vi "Teleop.vi"(10 "Match Info":T1={"Autonomous Elapsed Seconds"=0.0, "TeleOp Elapsed Seconds"=0.0, "Disabled Elapsed Seconds"=0.0, "Visited Autonomous"=FALSE, "Visited TeleOp"=FALSE, "Visited Disabled"=FALSE, "Autonomous Settings"={"Autonomous Style"=enum."Independent", "VI Refnum"=refnum}}, 11 "Call Context":T2) -> ()   [LabVIEW 2017]
doc: "This VI is called for each enabled TeleOp packet received from the DS. It is typically used to read from joysticks and other inputs and update I/O or setpoints for timed control loops. It should complete and return within 20 milliseconds or risk missing DS packets."
uses:
  <vilib>/Rock Robotics/WPI/DriverStation/WPI_DriverStationDerivedRobotMode.ctl
  <vilib>/Rock Robotics/WPI/DriverStation/WPI_DriverStationMatch Info.ctl
  Framework/Robot Global Data.vi
panel:
  out "Hardware Fault":bool
  out "Temperature Fault":bool
  out "Battery Voltage Fault":bool
  out "Current Faults":bool[](array[boolean])
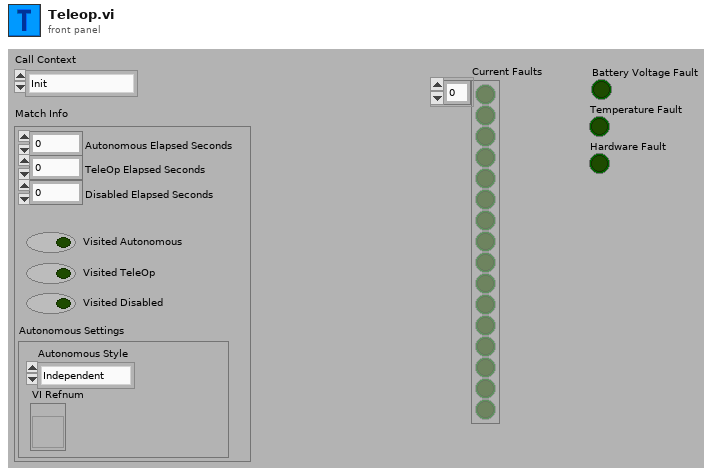
[diagram p1: front panel]
types:
  T1 = typedef "WPI_DriverStationMatch Info.ctl" = cluster{"Autonomous Elapsed Seconds":dbl, "TeleOp Elapsed Seconds":dbl, "Disabled Elapsed Seconds":dbl, "Visited Autonomous":bool, "Visited TeleOp":bool, "Visited Disabled":bool, "Autonomous Settings":cluster{"Autonomous Style":enum16{"Iterative", "Independent"}, "VI Refnum":refnum<vi>}}
  T2 = typedef "WPI_DriverStationDerivedRobotMode.ctl" = enum16{"Init", "Execute", "Stop"}
  T3 = enum16{"Normal", "Square", "Square with Rate", "Square Root", "Linear", "Exponential"}
  T4 = enum16{"Linear", "Square  Root", "Square", "n^x"}
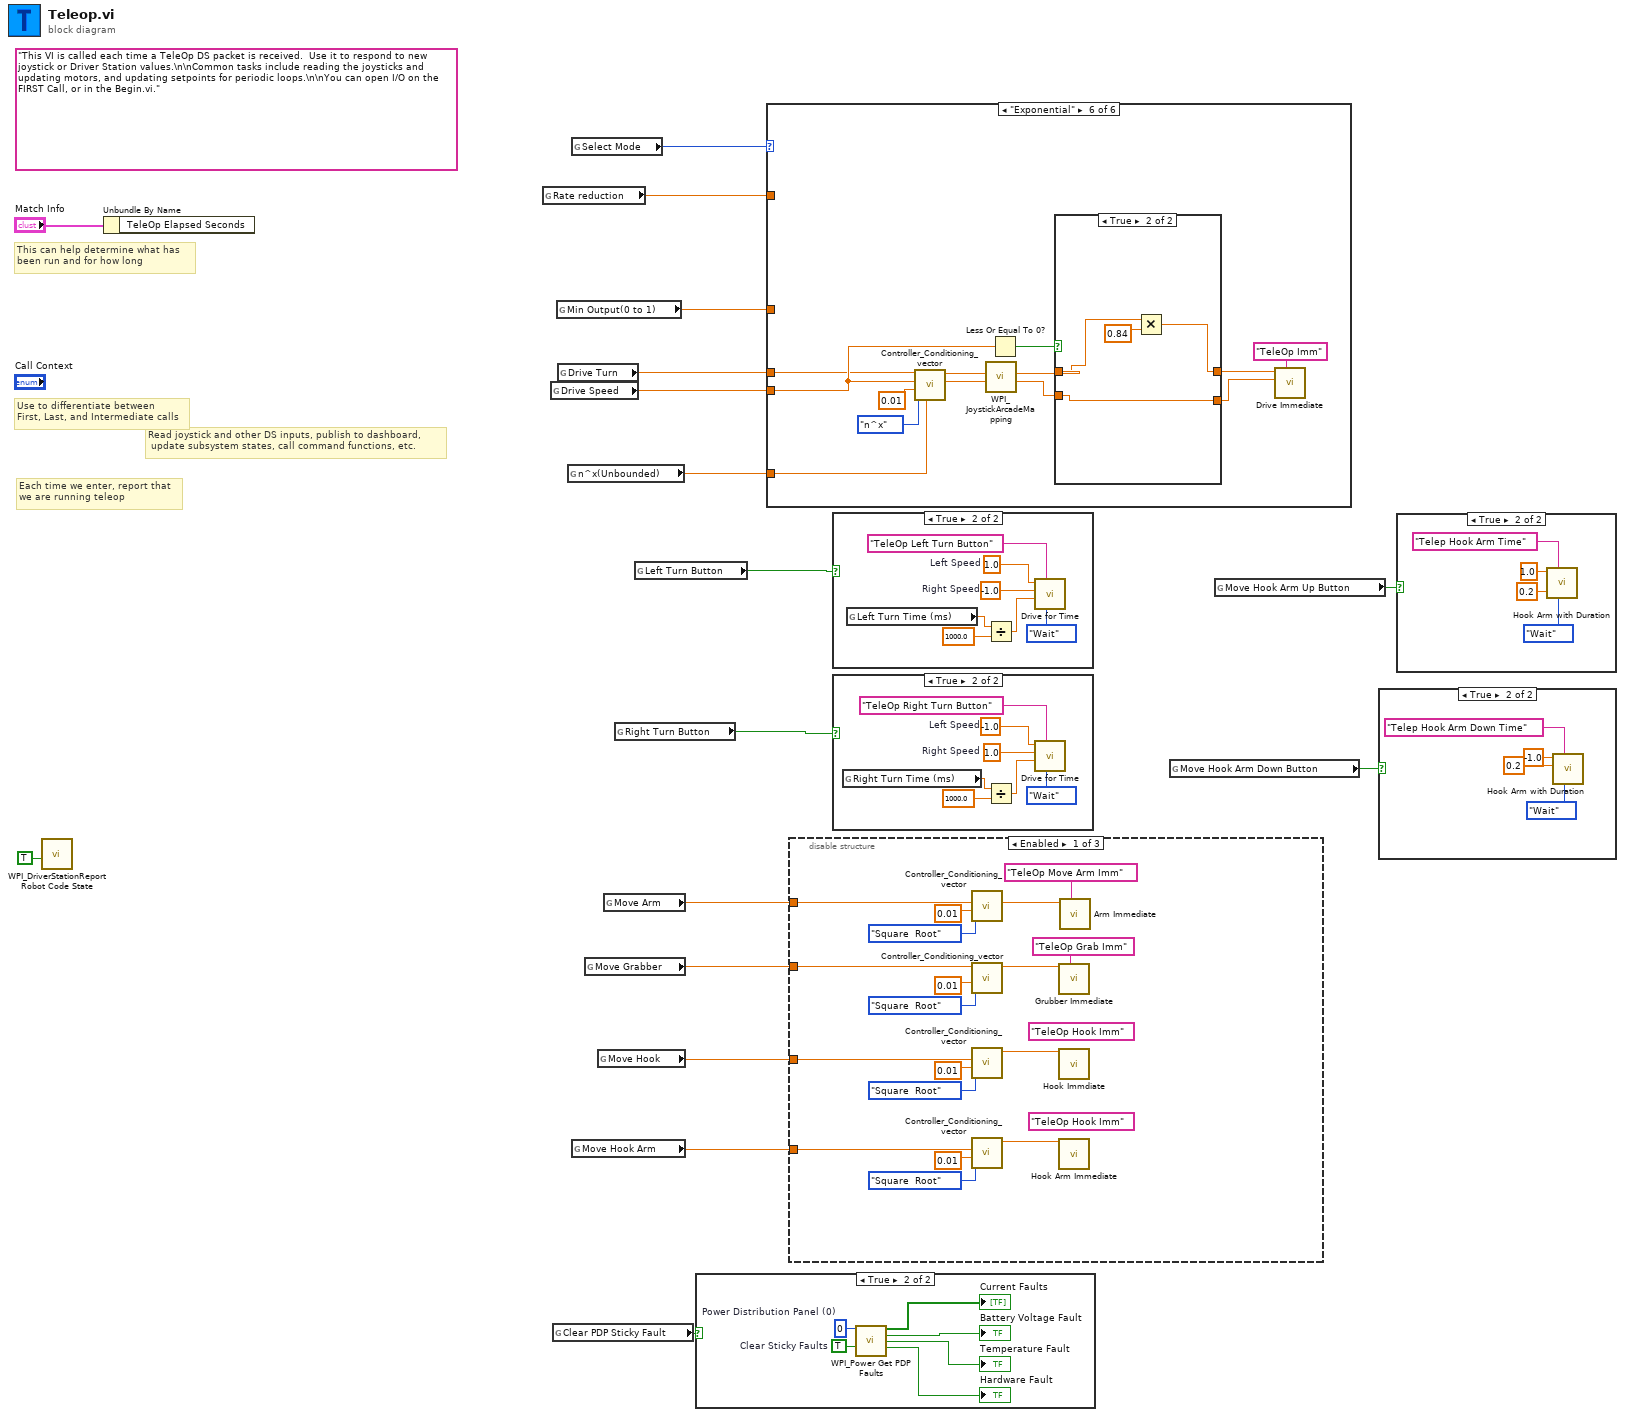
[diagram p0: block diagram]
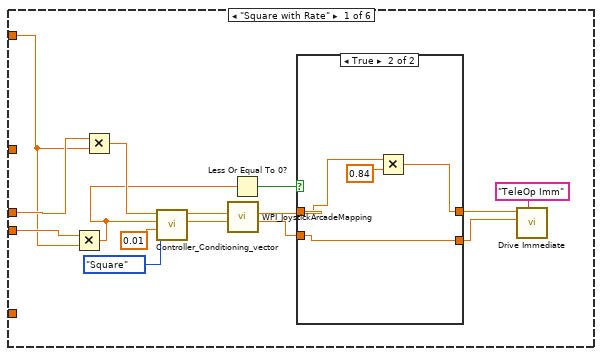
[diagram p7: hidden frame]
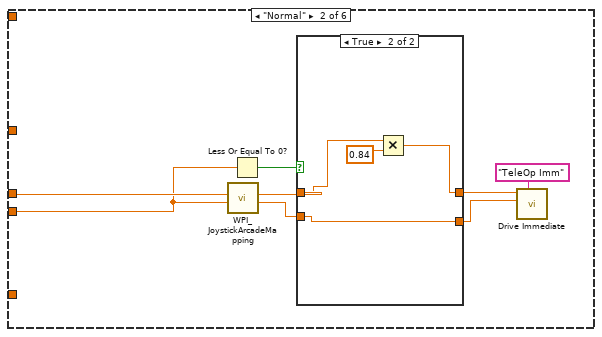
[diagram p9: hidden frame]
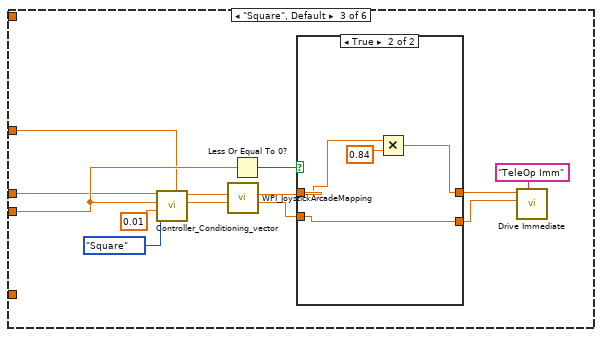
[diagram p11: hidden frame]
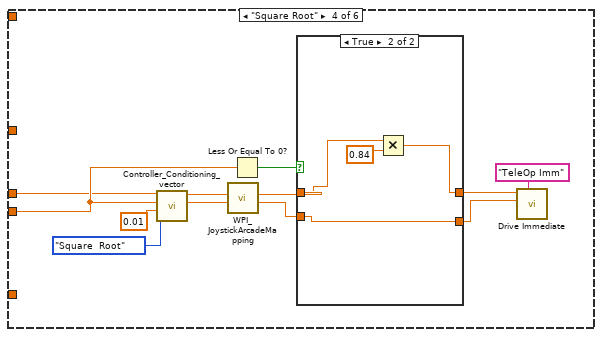
[diagram p13: hidden frame]
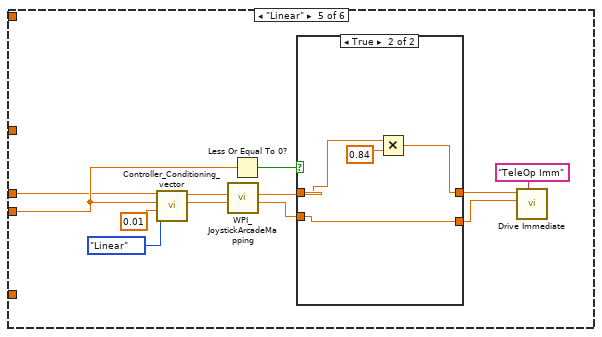
[diagram p15: hidden frame]
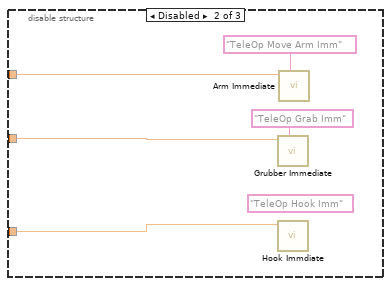
[diagram p18: hidden frame]
diagram:
  (unwired) "This VI is called each time a TeleOp DS packet is received.  Use it to respond to new joystick or Driver Station values.\n\nCommon tasks include reading the joysticks and updating motors, and updating setpoints for periodic loops.\n\nYou can open I/O on the FIRST Call, or in the Begin.vi."
  # "Read joystick and other DS inputs, publish to dashboard,\n update subsystem states, call command functions, etc."
  # "Each time we enter, report that\nwe are running teleop"
  # "Use to differentiate between\nFirst, Last, and Intermediate calls"
  # "This can help determine what has\nbeen run and for how long"
  n1 = call <vilib>:"WPI_DriverStationReport Robot Code State.vi"("TeleOp"=TRUE ("Autonomous")) -> ()  [unwired: 10 in, 1 out]
  n2 = Unbundle By Name("Match Info") -> ()  [unwired: 1 out]
  n3 = global read "Robot Global Data.vi" "Rate reduction"() -> (w12:dbl)
  n4 = global read "Robot Global Data.vi" "Drive Speed"() -> (w10:dbl)
  n5 = global read "Robot Global Data.vi" "Clear PDP Sticky Fault"() -> (w3:bool)
  n6 = global read "Robot Global Data.vi" "Min Output(0 to 1)"() -> (w14:dbl)
  n7 = global read "Robot Global Data.vi" "Drive Turn"() -> (w11:dbl)
  n8 = global read "Robot Global Data.vi" "n^x(Unbounded)"() -> (w13:dbl)
  n9 = global read "Robot Global Data.vi" "Select Mode"() -> (w15:T3)
  n10 = global read "Robot Global Data.vi" "Move Hook Arm"() -> (w4:dbl)
  n11 = global read "Robot Global Data.vi" "Move Grabber"() -> (w6:dbl)
  n12 = global read "Robot Global Data.vi" "Move Hook"() -> (w5:dbl)
  n13 = global read "Robot Global Data.vi" "Move Arm"() -> (w7:dbl)
  n14 = global read "Robot Global Data.vi" "Right Turn Button"() -> (w8:bool)
  n15 = global read "Robot Global Data.vi" "Left Turn Button"() -> (w9:bool)
  n16 = case shown="True" w3 {
    frame False {
    }
    frame True {
      w22 = TRUE  # Clear Sticky Faults
      w23 = u8 0  # Power Distribution Panel (0)
      n17 = call <vilib>:"WPI_Power Get PDP Faults.vi"("Power Distribution Panel (0)"=w23, "Clear Sticky Faults"=w22) -> ("Current Faults"=→"Current Faults":bool[], "Battery Voltage Fault"=→"Battery Voltage Fault":bool, "Temperature Fault"=→"Temperature Fault":bool, "Hardware Fault"=→"Hardware Fault":bool)  [unwired: 9 in, 1 out]
    }
  }
  n18 = case shown="\"Exponential\"" w15 {
    tunnel: w11 -> [w38 w46 w60 w78 w96 w115]
    tunnel: w10 -> [w37 w45 w61 w79 w97 w116]
    tunnel: w14 -> [_ _ w59 _ _ _]
    tunnel: w13 -> [_ _ _ _ _ w114]
    tunnel: w12 -> [w24 _ _ _ _ _]
    frame "Square with Rate" {
      n19 = Multiply(x=w37, y=w24) -> (x*y=w25:dbl)
      n20 = Multiply(x=w38, y=w24) -> (x*y=w26:dbl)
      n21 = call "Controller_Conditioning_vector.vi"("Enum"=T4."Square", "Dead Zone(0 to 1)"=0.01, "Y(-1 to 1)"=w25, "X(-1 to 1)"=w26) -> ("Y"=w27:dbl, "X"=w28:dbl)  [unwired: 4 in, 2 out]
      n22 = call <vilib>:"WPI_JoystickArcadeMapping.vi"("Y axis value"=w27, "X axis value"=w28) -> ("Right Motor Value"=w33:dbl, "Left Motor Value"=w34:dbl)  [unwired: 8 in]
      n23 = Less Or Equal To 0?(x=w25) -> (x <= 0?=w35:bool)
      n24 = case shown="True" w35 {
        tunnel: w34 -> [w39 w43]
        tunnel: [w39 w42] -> w32
        tunnel: w33 -> [w40 w41]
        tunnel: [w40 w41] -> w31
        frame False {
        }
        frame True {
          n25 = Multiply(x=w43, y=0.84) -> (x*y=w42:dbl)
        }
      }
      n26 = call "Drive Immediate.vi"("Description"="TeleOp Imm", "Right Setpoint"=w31, "Left Setpoint"=w32) -> ()  [unwired: 8 in, 1 out]
    }
    frame "Normal" {
      n27 = call <vilib>:"WPI_JoystickArcadeMapping.vi"("Y axis value"=w45, "X axis value"=w46) -> ("Right Motor Value"=w49:dbl, "Left Motor Value"=w50:dbl)  [unwired: 8 in]
      n28 = Less Or Equal To 0?(x=w45) -> (x <= 0?=w51:bool)
      n29 = case shown="True" w51 {
        tunnel: w50 -> [w53 w57]
        tunnel: [w53 w56] -> w48
        tunnel: w49 -> [w54 w55]
        tunnel: [w54 w55] -> w47
        frame False {
        }
        frame True {
          n30 = Multiply(x=w57, y=0.84) -> (x*y=w56:dbl)
        }
      }
      n31 = call "Drive Immediate.vi"("Description"="TeleOp Imm", "Right Setpoint"=w47, "Left Setpoint"=w48) -> ()  [unwired: 8 in, 1 out]
    }
    frame "Square", Default {
      n32 = call "Controller_Conditioning_vector.vi"("Min Output(0 to 1)"=w59, "Enum"=T4."Square", "Dead Zone(0 to 1)"=0.01, "Y(-1 to 1)"=w61, "X(-1 to 1)"=w60) -> ("Y"=w62:dbl, "X"=w63:dbl)  [unwired: 3 in, 2 out]
      n33 = call <vilib>:"WPI_JoystickArcadeMapping.vi"("Y axis value"=w62, "X axis value"=w63) -> ("Right Motor Value"=w68:dbl, "Left Motor Value"=w69:dbl)  [unwired: 8 in]
      n34 = Less Or Equal To 0?(x=w61) -> (x <= 0?=w70:bool)
      n35 = case shown="True" w70 {
        tunnel: w69 -> [w72 w76]
        tunnel: [w72 w75] -> w67
        tunnel: w68 -> [w73 w74]
        tunnel: [w73 w74] -> w66
        frame False {
        }
        frame True {
          n36 = Multiply(x=w76, y=0.84) -> (x*y=w75:dbl)
        }
      }
      n37 = call "Drive Immediate.vi"("Description"="TeleOp Imm", "Right Setpoint"=w66, "Left Setpoint"=w67) -> ()  [unwired: 8 in, 1 out]
    }
    frame "Square Root" {
      n38 = call "Controller_Conditioning_vector.vi"("Enum"=T4."Square  Root", "Dead Zone(0 to 1)"=0.01, "Y(-1 to 1)"=w79, "X(-1 to 1)"=w78) -> ("Y"=w80:dbl, "X"=w81:dbl)  [unwired: 4 in, 2 out]
      n39 = call <vilib>:"WPI_JoystickArcadeMapping.vi"("Y axis value"=w80, "X axis value"=w81) -> ("Right Motor Value"=w86:dbl, "Left Motor Value"=w87:dbl)  [unwired: 8 in]
      n40 = Less Or Equal To 0?(x=w79) -> (x <= 0?=w88:bool)
      n41 = case shown="True" w88 {
        tunnel: w87 -> [w90 w94]
        tunnel: [w90 w93] -> w85
        tunnel: w86 -> [w91 w92]
        tunnel: [w91 w92] -> w84
        frame False {
        }
        frame True {
          n42 = Multiply(x=w94, y=0.84) -> (x*y=w93:dbl)
        }
      }
      n43 = call "Drive Immediate.vi"("Description"="TeleOp Imm", "Right Setpoint"=w84, "Left Setpoint"=w85) -> ()  [unwired: 8 in, 1 out]
    }
    frame "Linear" {
      n44 = call "Controller_Conditioning_vector.vi"("Enum"=T4."Linear", "Dead Zone(0 to 1)"=0.01, "Y(-1 to 1)"=w97, "X(-1 to 1)"=w96) -> ("Y"=w98:dbl, "X"=w99:dbl)  [unwired: 4 in, 2 out]
      n45 = call <vilib>:"WPI_JoystickArcadeMapping.vi"("Y axis value"=w98, "X axis value"=w99) -> ("Right Motor Value"=w104:dbl, "Left Motor Value"=w105:dbl)  [unwired: 8 in]
      n46 = Less Or Equal To 0?(x=w97) -> (x <= 0?=w106:bool)
      n47 = case shown="True" w106 {
        tunnel: w105 -> [w108 w112]
        tunnel: [w108 w111] -> w103
        tunnel: w104 -> [w109 w110]
        tunnel: [w109 w110] -> w102
        frame False {
        }
        frame True {
          n48 = Multiply(x=w112, y=0.84) -> (x*y=w111:dbl)
        }
      }
      n49 = call "Drive Immediate.vi"("Description"="TeleOp Imm", "Right Setpoint"=w102, "Left Setpoint"=w103) -> ()  [unwired: 8 in, 1 out]
    }
    frame "Exponential" {
      n50 = call "Controller_Conditioning_vector.vi"("n^x(Unbounded)"=w114, "Enum"=T4."n^x", "Dead Zone(0 to 1)"=0.01, "Y(-1 to 1)"=w116, "X(-1 to 1)"=w115) -> ("Y"=w117:dbl, "X"=w118:dbl)  [unwired: 3 in, 2 out]
      n51 = call <vilib>:"WPI_JoystickArcadeMapping.vi"("Y axis value"=w117, "X axis value"=w118) -> ("Right Motor Value"=w123:dbl, "Left Motor Value"=w124:dbl)  [unwired: 8 in]
      n52 = Less Or Equal To 0?(x=w116) -> (x <= 0?=w125:bool)
      n53 = case shown="True" w125 {
        tunnel: w124 -> [w127 w131]
        tunnel: [w127 w130] -> w122
        tunnel: w123 -> [w128 w129]
        tunnel: [w128 w129] -> w121
        frame False {
        }
        frame True {
          n54 = Multiply(x=w131, y=0.84) -> (x*y=w130:dbl)
        }
      }
      n55 = call "Drive Immediate.vi"("Description"="TeleOp Imm", "Right Setpoint"=w121, "Left Setpoint"=w122) -> ()  [unwired: 8 in, 1 out]
    }
  }
  n56 = disable-structure shown="Enabled" {
    disable-tunnel: w7 -> [w145 w153 _]
    disable-tunnel: w6 -> [w144 w152 _]
    disable-tunnel: w5 -> [w137 w151 _]
    disable-tunnel: w4 -> [w136 _ _]
    frame Enabled {
      (unwired) "TeleOp Hook Imm" ("Description")
      (unwired) "TeleOp Hook Imm" ("Description")
      n57 = call "Controller_Conditioning_vector.vi"("Enum"=T4."Square  Root", "Dead Zone(0 to 1)"=0.01, "Y(-1 to 1)"=w145) -> ("Y"=w148:dbl)  [unwired: 5 in, 3 out]
      n58 = call "Controller_Conditioning_vector.vi"("Enum"=T4."Square  Root", "Dead Zone(0 to 1)"=0.01, "X(-1 to 1)"=w144) -> ("X"=w143:dbl)  [unwired: 5 in, 3 out]
      n59 = call "Controller_Conditioning_vector.vi"("Enum"=T4."Square  Root", "Dead Zone(0 to 1)"=0.01, "Y(-1 to 1)"=w137) -> ("X"=w140:dbl)  [unwired: 5 in, 3 out]
      n60 = call "Controller_Conditioning_vector.vi"("Enum"=T4."Square  Root", "Dead Zone(0 to 1)"=0.01, "Y(-1 to 1)"=w136) -> ("X"=w133:dbl)  [unwired: 5 in, 3 out]
      n61 = call "Grubber Immediate.vi"("Description"="TeleOp Grab Imm", "Setpoint"=w143) -> ()  [unwired: 9 in, 1 out]
      n62 = call "Hook Immdiate.vi"("Setpoint"=w140) -> ()  [unwired: 10 in, 1 out]
      n63 = call "Hook Arm Immediate.vi"("Setpoint"=w133) -> ()  [unwired: 10 in, 1 out]
      n64 = call "Arm Immediate.vi"("Description"="TeleOp Move Arm Imm", "Setpoint"=w148) -> ()  [unwired: 9 in, 1 out]
    }
    frame Disabled {
      (unwired) "TeleOp Hook Imm" ("Description")
      n65 = call "Grubber Immediate.vi"("Description"="TeleOp Grab Imm", "Setpoint"=w152) -> ()  [unwired: 9 in, 1 out]
      n66 = call "Hook Immdiate.vi"("Setpoint"=w151) -> ()  [unwired: 10 in, 1 out]
      n67 = call "Arm Immediate.vi"("Description"="TeleOp Move Arm Imm", "Setpoint"=w153) -> ()  [unwired: 9 in, 1 out]
    }
    frame Disabled {
    }
  }
  n68 = case shown="True" w9 {
    frame False {
    }
    frame True {
      w157 = -1.0  # Right Speed
      w156 = 1.0  # Left Speed
      n69 = global read "Robot Global Data.vi" "Left Turn Time (ms)"() -> (w161:dbl)
      n70 = Divide(x=w161, y=1000.0) -> (x/y=w162:dbl)
      n71 = call "Drive for Time.vi"("Synchronization"=enum16{"Start", "Wait"}."Wait" ("Synchronication"), "Description"="TeleOp Left Turn Button", "Seconds"=w162, "Right Speed"=w157, "Left Speed"=w156) -> ()  [unwired: 5 in, 2 out]
    }
  }
  n72 = case shown="True" w8 {
    frame False {
    }
    frame True {
      w164 = 1.0  # Right Speed
      w163 = -1.0  # Left Speed
      n73 = global read "Robot Global Data.vi" "Right Turn Time (ms)"() -> (w168:dbl)
      n74 = Divide(x=w168, y=1000.0) -> (x/y=w169:dbl)
      n75 = call "Drive for Time.vi"("Synchronization"=enum16{"Start", "Wait"}."Wait" ("Synchronication"), "Description"="TeleOp Right Turn Button", "Seconds"=w169, "Right Speed"=w164, "Left Speed"=w163) -> ()  [unwired: 5 in, 2 out]
    }
  }
  n76 = global read "Robot Global Data.vi" "Move Hook Arm Down Button"() -> (w1:bool)
  n77 = global read "Robot Global Data.vi" "Move Hook Arm Up Button"() -> (w2:bool)
  n78 = case shown="True" w1 {
    frame False {
    }
    frame True {
      n79 = call "Hook Arm with Duration.vi"("Synchronization"=enum16{"Start", "Wait"}."Wait", "Description"="Telep Hook Arm Down Time", "Duration (s)"=0.2, "Setpoint"=-1.0) -> ()  [unwired: 7 in, 1 out]
    }
  }
  n80 = case shown="True" w2 {
    frame False {
    }
    frame True {
      n81 = call "Hook Arm with Duration.vi"("Synchronization"=enum16{"Start", "Wait"}."Wait", "Description"="Telep Hook Arm Time", "Duration (s)"=0.2, "Setpoint"=1.0) -> ()  [unwired: 7 in, 1 out]
    }
  }
